vi "ClassPanel.vi"(8 "error in (no error)":errorcluster caption="entrée d'erreur (pas d'erreur)", 11 "AppliedMotionDrive.lvclass":refnum<class "AppliedMotionDrive.lvclass">) -> (0 "error out":errorcluster caption="sortie d'erreur", 3 "AppliedMotionDrive.lvclass Out":refnum<class "AppliedMotionDrive.lvclass">)   [LabVIEW 2019, in "AppliedMotionDrive.lvclass"]
uses:
  AppliedMotionDrive.lvclass
  C:/Programmes Labview/LabscanV1A/DevicesClass/BaseDevice/BaseDevice.lvclass
  AppliedMotionDrive.lvclass/AppliedMotionDrive.ctl
  BaseDevice/Accessor/GetClassEvent.vi
panel:
  out "InstrName":string
  out "CCW Limit":bool
  out "CW Limit":bool
  in  "Stop Move":bool
  in  "Position(Units)":dbl caption="Position(mm)"
  in  "Stop":bool
  out "Init Program":bool
  # "this MUST labeled with class name"
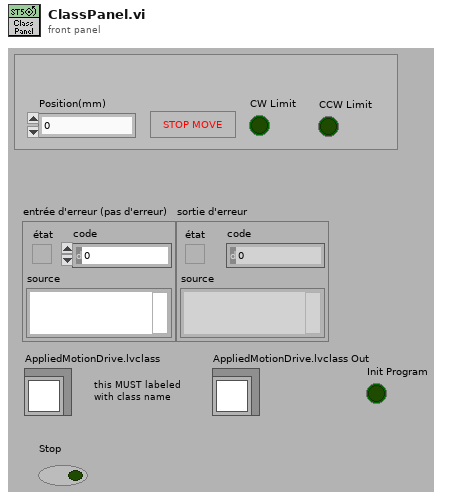
[diagram p1: front panel]
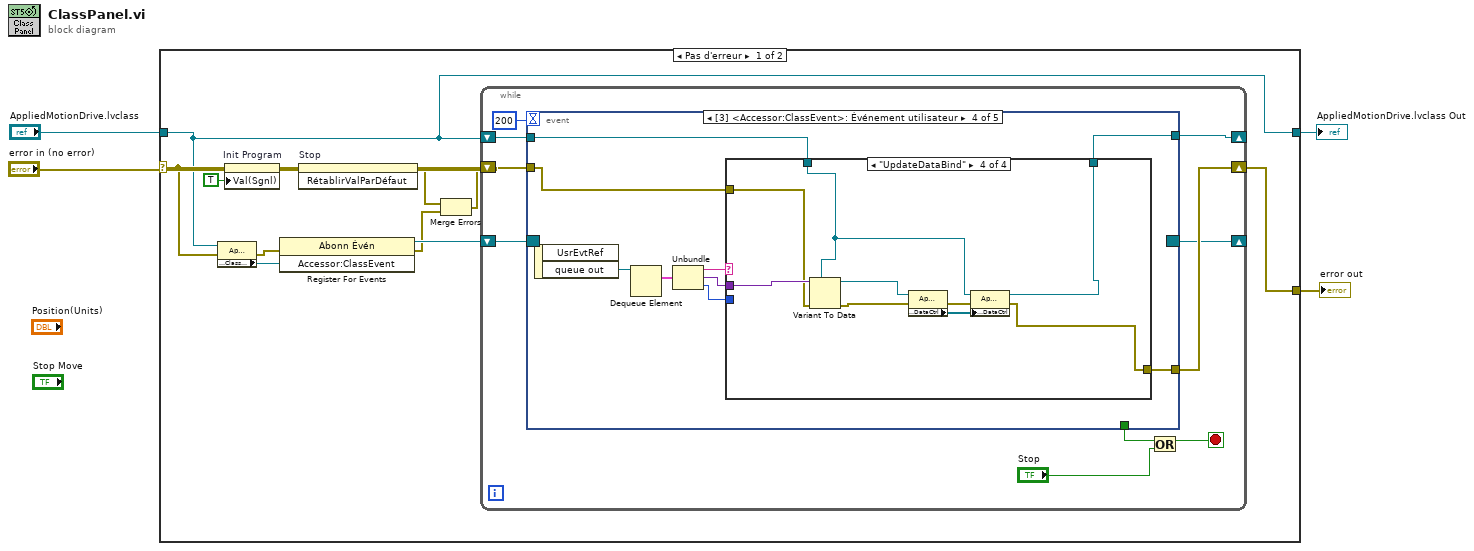
[diagram p0: block diagram]
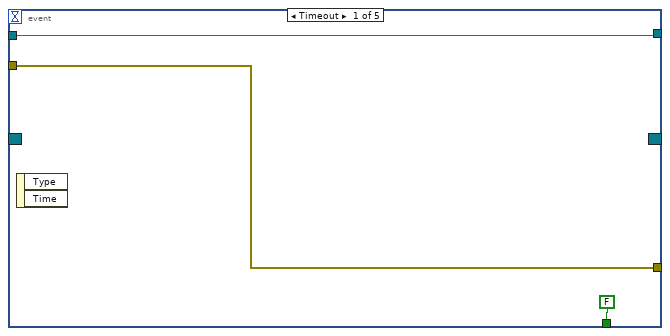
[diagram p2: hidden frame]
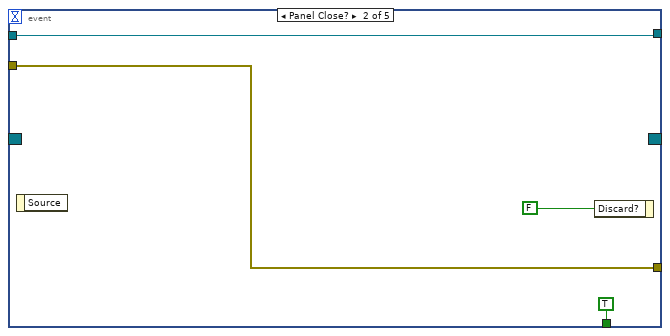
[diagram p3: hidden frame]
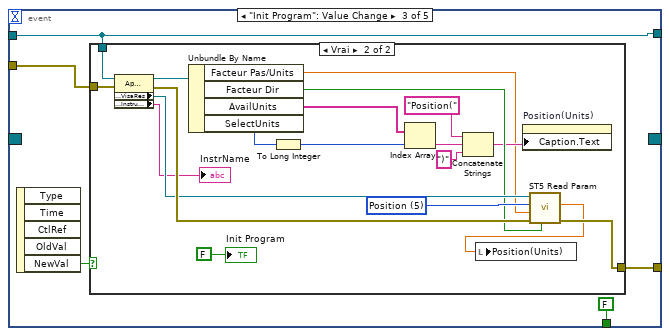
[diagram p4: hidden frame]
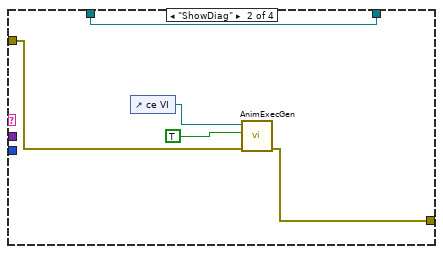
[diagram p7: hidden frame]
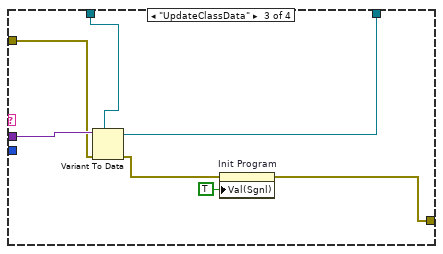
[diagram p8: hidden frame]
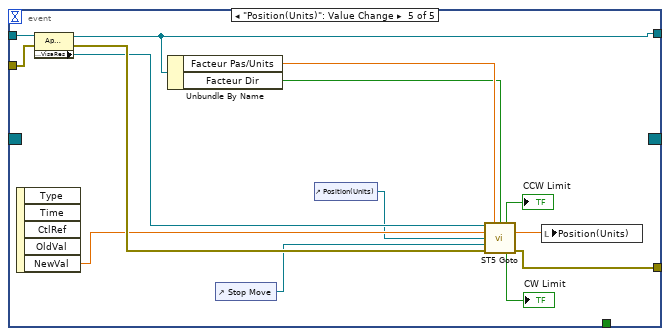
[diagram p9: hidden frame]
diagram:
  n1 = case shown="Pas d'erreur" "error in (no error)" {
    selector: "error in (no error)" -> [w5 w105]
    tunnel: [w15 w105] -> w3
    tunnel: "AppliedMotionDrive.lvclass" -> [w6 w104]
    tunnel: [w6 w104] -> w1
    frame No Error {
      n2 = property class="AppliedMotionDrive.lvclass"(reference=w6, error in=w5) -> (error out=w10:errorcluster, "Accessor:ClassEvent"=w11:refnum<user-event>)  [unwired: 1 out]
      n3 = property on="Init Program" class="Bool (strict)"(error in=w5, "Val(Sgnl)"=TRUE ("Valeur (Signalisation)")) -> (error out=w13:errorcluster)  [unwired: 1 in, 1 out]
      n4 = register-events(error in=w10, w11) -> (reference out=w12:refnum<event-registration>, error out=w9:errorcluster)  [unwired: 1 in]
      n5 = invoke on="Stop" class="Bool (strict)" method="RétablirValParDéfaut"(error in=w13) -> (error out=w8:errorcluster)  [unwired: 2 in, 2 out]
      n6 = Merge Errors(w8, w9) -> (w7:errorcluster)
      n7 = while {
        shift-right: [w23] -> w15
        shift-left: w7 -> [w24]
        shift-right: [w16] -> _
        shift-left: w6 -> [w17]
        shift-right: [w18] -> _
        shift-left: w12 -> [w19]
        stop <- w21 stop-if-true
        n8 = event shown="[3] <Accessor:ClassEvent>: Événement utilisateur" {
          selector: w19 -> [_ _ _ _ _]
          dyn-events: [_ _ _ _ _] -> w18
          timeout: 200 -> [_ _ _ _ _]
          tunnel: w24 -> [w27 w30 w36 w66 w103]
          tunnel: [w27 w30 w35 w58 w98] -> w23
          tunnel: [FALSE TRUE FALSE _ _] -> w22
          tunnel: w17 -> [w26 w29 w33 w60 w94]
          tunnel: [w26 w29 w33 w59 w93] -> w16
          event Timeout {
            n9 = event-data() -> ()  [unwired: 1 in, 2 out]
          }
          event Panel Close? {
            n10 = event-data() -> ()  [unwired: 1 in, 1 out]
            n11 = event-data("Discard?"=FALSE ("Rejeter ?")) -> ()  [unwired: 1 in, 1 out]
          }
          event "Init Program": Value Change {
            n12 = event-data() -> ("NewVal"=w37:bool)  [unwired: 1 in, 4 out]
            n13 = case shown="Vrai" w37 {
              tunnel: w36 -> [w38 w55]
              tunnel: [w38 w50] -> w35
              tunnel: w33 -> [_ w40]
              frame False {
              }
              frame True {
                w56 = u16 5 items=["All", "Velocity", "Acceleration", "Deceleration", "Max Acceleration", "Position", "Step/Rev", "Alarm Code", "Status"] ("Parameters")
                n14 = property class="AppliedMotionDrive.lvclass"(reference=w40, error in=w55) -> (reference out=w53:refnum<class "AppliedMotionDrive.lvclass">, error out=w54:errorcluster, "Accessor:VisaRes"=w52:refnum<visa-resource-name>, "Accessor:InstrumentName"=→"InstrName":string)
                n15 = Unbundle By Name(w53) -> ("Facteur Pas/Units"=w39:dbl, "Facteur Dir"=w51:bool, "AvailUnits"=w47:string[], "SelectUnits"=w46:u8)
                n16 = To Long Integer(number=w46) -> (32bit integer=w41:i32)
                n17 = Index Array(array=w47, index=w41) -> (element=w45:string)
                n18 = Concatenate Strings("Position(" ("chaîne"), w45, ")" ("expression régulière")) -> (w43:string)
                n19 = property on="Position(Units)" class="NumNb (strict)"("Caption.Text"=w43) -> ()  [unwired: 2 in, 2 out]
                n20 = call <userlib>:"ST5 Read Param.vi"("Facteur Dir"=w51, "error in (no error)"=w54, "Facteur Pas"=w39, "Parameters"=w56, "Port COM"=w52) -> ("error out"=w50:errorcluster, "Position"=w49:dbl)  [unwired: 5 out]
                n21 = local write "Position(Units)"(w49) -> ()
                "Init Program" <- FALSE
              }
            }
          }
          event User Event {
            n22 = event-data() -> ("queue out"=w65:refnum<queue>)  [unwired: 1 in, 1 out]
            n23 = Dequeue Element(queue=w65) -> (element=w64:cluster{"Message":string, "Data":variant, i32})  [unwired: 2 in, 3 out]
            n24 = Unbundle(w64) -> ("Message"=w63:string, "Data"=w61:variant, w62:i32)
            n25 = case shown="\"UpdateDataBind\"" w63 {
              tunnel: w66 -> [w67 w70 w77 w88]
              tunnel: w61 -> [_ _ w80 w89]
              tunnel: w62 -> [_ _ _ _]
              tunnel: w60 -> [w68 w71 w79 w84]
              tunnel: [w68 w71 w78 w81] -> w59
              tunnel: [w67 w69 w74 w82] -> w58
              frame Default {
              }
              frame "ShowDiag" {
                n26 = control-ref of="ce VI"() -> (w72:refnum<vi>)
                n27 = call <userlib>:"AnimExecGen.vi"("ErrorIn(No Error)"=w70, "Animer l'exécution ?"=TRUE, "ViRef"=w72) -> ("sortie d'erreur"=w69:errorcluster)  [unwired: 8 in]
              }
              frame "UpdateClassData" {
                n28 = Variant To Data(error in=w77, type=w79, Variant=w80) -> (data=w78:refnum<class "AppliedMotionDrive.lvclass">, error out=w75:errorcluster)
                n29 = property on="Init Program" class="Bool (strict)"(error in=w75, "Val(Sgnl)"=TRUE ("Valeur (Signalisation)")) -> (error out=w74:errorcluster)  [unwired: 1 in, 1 out]
              }
              frame "UpdateDataBind" {
                n30 = Variant To Data(error in=w88, type=w84, Variant=w89) -> (data=w85:refnum<class "AppliedMotionDrive.lvclass">, error out=w83:errorcluster)
                n31 = property class="AppliedMotionDrive.lvclass"(reference=w85, error in=w83) -> (error out=w87:errorcluster, "Accessor:DataCtrl"=w86:refnum<vi>[])  [unwired: 1 out]
                n32 = property class="AppliedMotionDrive.lvclass"(reference=w84, error in=w87, "Accessor:DataCtrl"=w86) -> (reference out=w81:refnum<class "AppliedMotionDrive.lvclass">, error out=w82:errorcluster)
              }
            }
          }
          event "Position(Units)": Value Change {
            n33 = event-data() -> ("NewVal"=w100:dbl)  [unwired: 1 in, 4 out]
            n34 = property class="AppliedMotionDrive.lvclass"(reference=w94, error in=w103) -> (reference out=w93:refnum<class "AppliedMotionDrive.lvclass">, error out=w102:errorcluster, "Accessor:VisaRes"=w101:refnum<visa-resource-name>)
            n35 = Unbundle By Name(w93) -> ("Facteur Pas/Units"=w97:dbl, "Facteur Dir"=w96:bool)
            n36 = control-ref of="Stop Move"() -> (w95:refnum<vi>)
            n37 = control-ref of="Position(Units)"() -> (w90:refnum<vi>)
            n38 = call <userlib>:"ST5 Goto.vi"("Port COM"=w101, "Facteur Pas"=w97, "Facteur Dir"=w96, "Position"=w100, "PositionRef"=w90, "Ext Stop Ref"=w95, "error in (no error)"=w102) -> ("CCW Limit"=→"CCW Limit":bool, "Position Out"=w99:dbl, "CW Limit"=→"CW Limit":bool, "error out"=w98:errorcluster)  [unwired: 2 in, 3 out]
            n39 = local write "Position(Units)"(w99) -> ()
          }
        }
        n40 = Or(x=w22, y="Stop") -> (x .or. y?=w21:bool)
      }
    }
    frame Error {
    }
  }
  "error out" <- w3
  "AppliedMotionDrive.lvclass Out" <- w1
